vi "Vision Tracking.vi"(8 "error in (no error)":errorcluster, 11 "Ideal Target Height (in)":i32) -> (2 "Distance (ft)":dbl, 3 "X-Value of Target (px)":dbl)   [LabVIEW 2016]
uses:
  <vilib>/Rock Robotics/WPI/Camera/WPI_CameraSettings Read MJPG.ctl
  <vilib>/Rock Robotics/WPI/Camera/WPI_CameraImageSize.ctl
  2017 Robot Project/Vision Support Code/Camera Types.ctl
  <vilib>/Rock Robotics/WPI/Camera/WPI_CameraExposure Values.ctl
  <vilib>/Rock Robotics/WPI/Camera/WPI_CameraWhite Balance Values.ctl
  <vilib>/vision/NI_Vision_Development_Module.lvlib
panel:
  in  "Line Border":cluster{"Top":dbl, "Bottom":dbl}={"Top"=6.0, "Bottom"=1.0}
  in  "Use Calibration":bool=TRUE
  out "Instructions:":string="Use Source to load image files from a directory, or use a USB or IP camera connected to your laptop. Use Camera Settings 1 and 2 to achieve a dark image with bright and colorful stripes.\nLED Color can encoded as HSL or related color modes. Calibrate to the same color as the strips being reflected to the camera.\nClick and draw a line in Original Image to auto-calibrate the LED Color. You may want to widen and tweak Sat and Val by hand.\nThe Annotate button affects drawing a rectangle around the stripes and labeling it with a distance in ft. Distance relies on knowing the Camera Type and lens calibration (it looks up the lens view angle).\n\nAdjust Score Cutoff to make the code more or less picky. If the color is not very unique, you may need to increase the number of particles considered. The diagram uses a Size Limit to ignore colored things that are too small. You may need to adjust it if you are targetting from far away.\n\nResults give you the distance to the target, the center and box in a normalized (-1 to 1) and pixel coordinates.\n\nBe sure to read about setting camera exposure and brightness to help simplify your image and acquire color saturated images.\n\nThere are lots of comments on the diagram to explain the code."
  in  "Color Mode":u16(ring)=3 items=["RGB", "HSL", "HSV", "HSI"]
  in  "Particles":dbl=5.0
  in  "Score Cutoff %":dbl=70.0
  in  "Std Devs for Calibration":cluster{"H":dbl, "S":dbl, "V":dbl}={"H"=4.0, "S"=6.0, "V"=6.0}
  in  "Camera Type":T1=enum."MS HD3000 square"
  in  "image files":string[](array[string])
  out "Results":T2 {"Score" format="%#_3g"; "Pixels"."Rectangle"."Numeric 5" format="%#_3g"; "Pixels"."Rectangle"."Numeric 3" format="%#_3g"; "Pixels"."Rectangle"."Numeric 2" format="%#_3g"; "Pixels"."Rectangle"."Numeric" format="%#_3g"; "Normalized"."Rectangle"."Numeric 5" format="%#_2g"; "Normalized"."Rectangle"."Numeric 3" format="%#_2g"; "Normalized"."Rectangle"."Numeric 2" format="%#_2g"; "Normalized"."Rectangle"."Numeric" format="%#_2g"; "Normalized"."Center"."?" format="%#_3g"; "Normalized"."Center"."?" format="%#_3g"; "Distance (ft)" format="%#_3g"}
  in  "Source":enum32{"Files", "Camera"}(tab)
  in  "Images":i32(listbox)
  in  "Folder Location":path=path "C:/Program Files (x86)/National Instruments/LabVIEW 2016/examples/FRC/roboRIO/Vision/2017 Vision Example/Sample Images/LED Boiler"
  in  "Camera Settings":T3={"fps"=20, "compression"=30, "Image Size"=enum."320x240", "Config Shown"=FALSE}
  in  "Camera Address":string="USB 1"
  in  "Camera Settings 2":T7={"Exposure"=enum."Auto", "Exposure (%)"=50.0, "Brightness"=50, "White Balance"=enum."Auto", "Color Temp (K)"=0.0} {"Brightness" min=0 max=100}
  in  "Annotate":bool=TRUE
  out "Qualified Particles":i32
  in  "LED Color":T8={"Hue"={107.81818389892578, 139.81818389892578}, "Sat"={176.07142857142858, 255.0}, "Val"={40.53571428571429, 255.0}} {"Hue" scale=0.0..255.0 scale format="%#_3g"}
  out "Mask":T9(plugin-control)
  out "Original Image":T9(plugin-control)
  # "Legend:\n    Rectangle\n       Green - Good target, distance ft\n       Red - Bad target\n    Orange Text - Score in %"
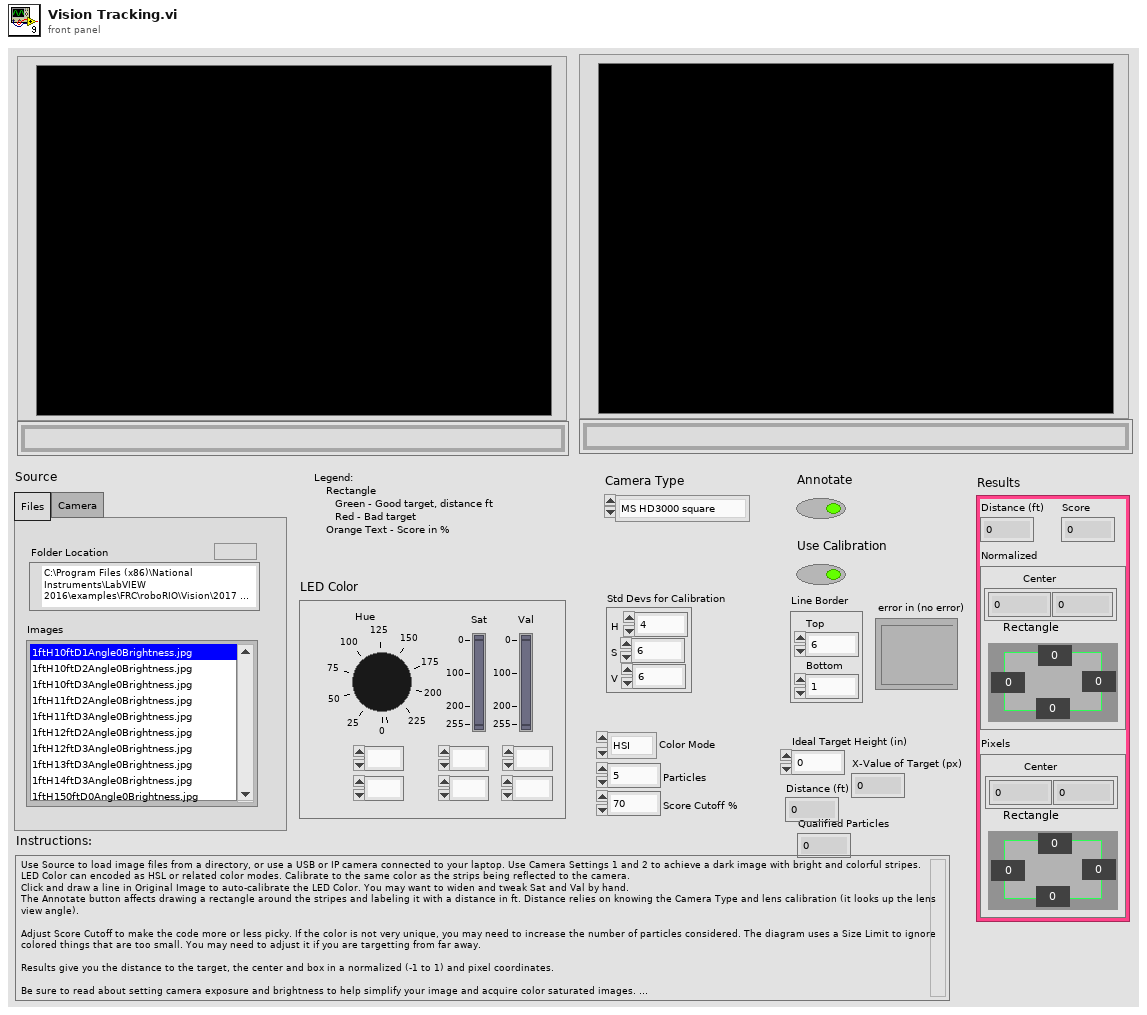
[diagram p1: front panel]
types:
  T1 = typedef "Camera Types.ctl" = enum16{"206", "1011", "1013", "MS HD3000 square", "MS HD3000 640x480"}
  T2 = cluster{"Distance (ft)":dbl, "Score":dbl, "Normalized":cluster{"Center":cluster{dbl, dbl}, "Rectangle":cluster{"Numeric":dbl, "Numeric 2":dbl, "Numeric 3":dbl, "Numeric 5":dbl}}, "Pixels":cluster{"Center":cluster{dbl, dbl}, "Rectangle":cluster{"Numeric":dbl, "Numeric 2":dbl, "Numeric 3":dbl, "Numeric 5":dbl}}}
  T3 = typedef "WPI_CameraSettings Read MJPG.ctl" = cluster{"fps":i32, "compression":i32, "Image Size":T4, "Config Shown":bool}
  T4 = typedef "WPI_CameraImageSize.ctl" = enum16{"640x480", "320x240", "160x120", "Custom"}
  T5 = typedef "WPI_CameraExposure Values.ctl" = enum16{"Auto", "Flicker-free 50 Hz", "Flicker-free 60 Hz", "Hold current", "Custom"}
  T6 = typedef "WPI_CameraWhite Balance Values.ctl" = enum16{"Auto", "Fixed indoor", "Fixed outdoor 1", "Fixed outdoor 2", "Fixed fluorescent 1", "Fixed fluorescent 2", "Hold current", "Custom"}
  T7 = cluster{"Exposure":T5, "Exposure (%)":dbl, "Brightness":i32, "White Balance":T6, "Color Temp (K)":dbl}
  T8 = cluster{"Hue":cluster{dbl, dbl}, "Sat":cluster{dbl, dbl}, "Val":cluster{dbl, dbl}}
  T9 = typedef "IMAQ Image.ctl" = refnum<image>
  T10 = typedef "Image Type" = u32
  T11 = typedef "Particle Parameters" = i32
  T12 = cluster{cluster{dbl, dbl}, cluster{dbl, dbl}, cluster{dbl, dbl}}
  T13 = cluster{"Left":dbl, "Top":dbl, "Right":dbl, "Bottom":dbl}
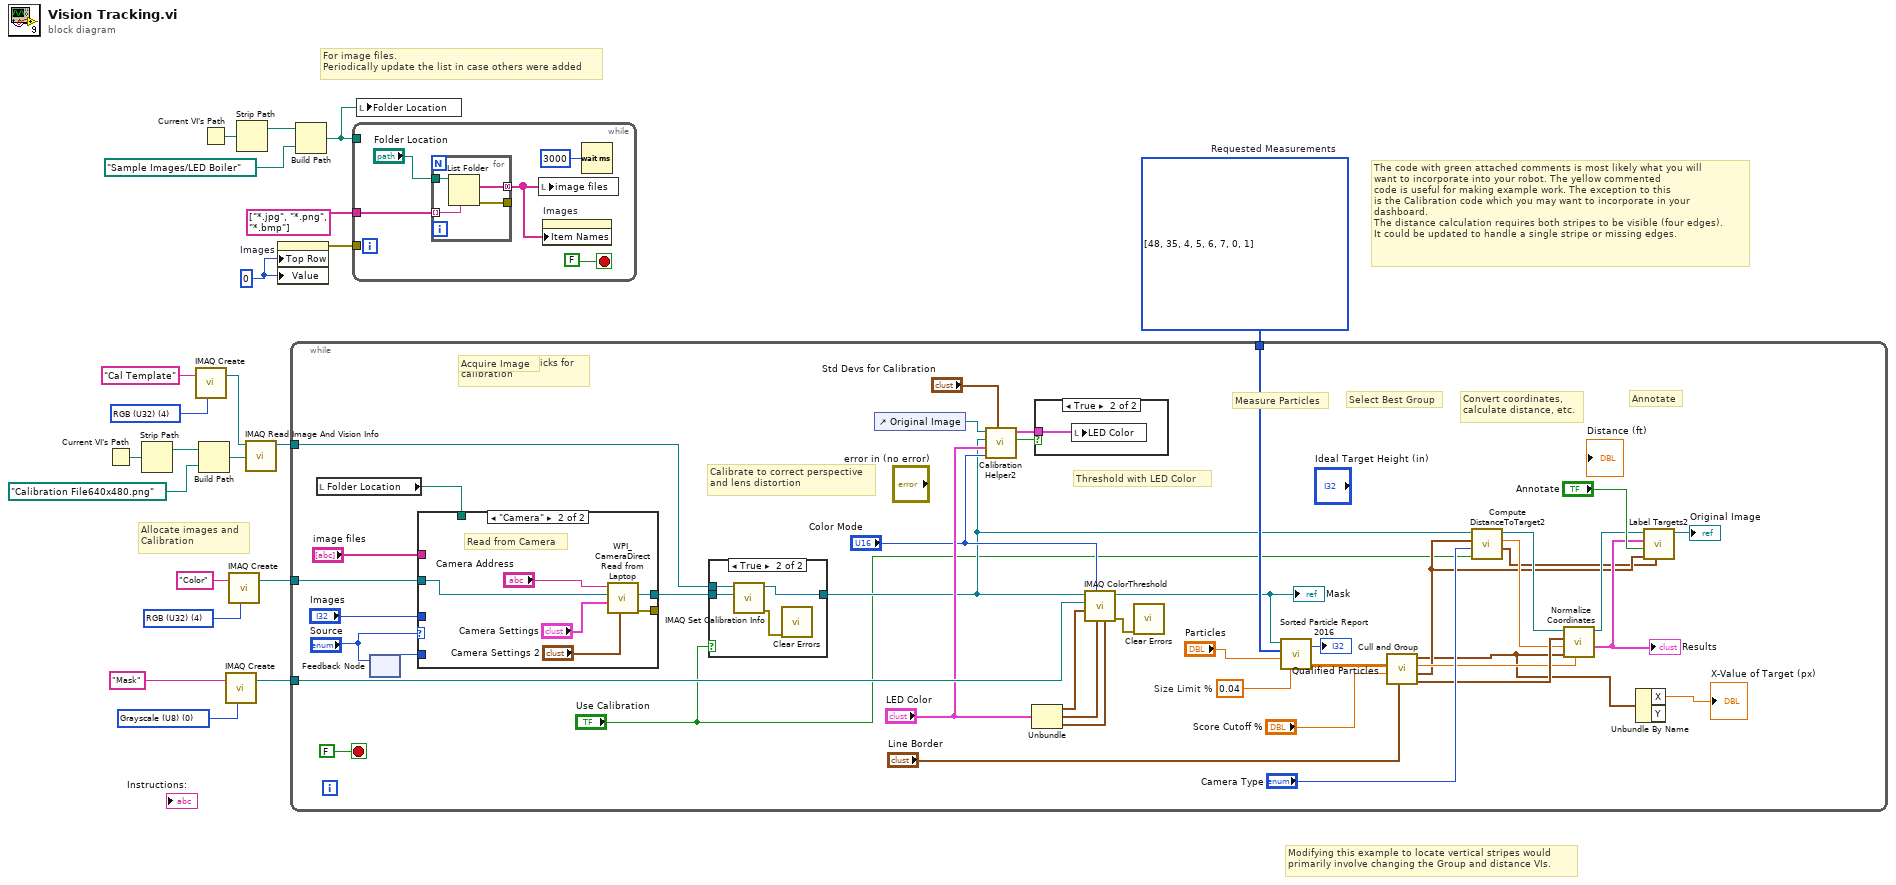
[diagram p0: block diagram]
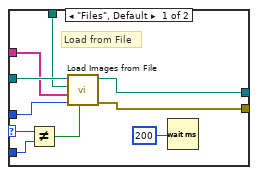
[diagram p4: hidden frame]
diagram:
  w8 = T10 4 items=["Grayscale (U8)", "Grayscale (I16)", "Grayscale (SGL)", "Complex (CSG)", "RGB (U32)", "HSL (U32)", "RGB (U64)", "Grayscale (U16)"] ("Image Type")
  w11 = u32 0 ("milliseconds to wait")
  w17 = T11[] [48, 35, 4, 5, 6, 7, 0, 1] items=["Center of Mass X", "Center of Mass Y", "First Pixel X", "First Pixel Y", "Bounding Rect Left", "Bounding Rect Top", "Bounding Rect Right", "Bounding Rect Bottom", "Max Feret Diameter Start X", "Max Feret Diameter Start Y", "Max Feret Diameter End X", "Max Feret Diameter End Y", "Max Horiz. Segment Length Left", "Max Horiz. Segment Length Right", "Max Horiz. Segment Length Row", "-", "Bounding Rect Width", "Bounding Rect Height", "Bounding Rect Diagonal", "Perimeter", "Convex Hull Perimeter", "Holes' Perimeter", "Max Feret Diameter", "Equivalent Ellipse Major Axis", "Equivalent Ellipse Minor Axis", "Equivalent Ellipse Minor Axis (Feret)", "Equivalent Rect Long Side", "Equivalent Rect Short Side", "Equivalent Rect Diagonal", "Equivalent Rect Short Side (Feret)", "Average Horiz. Segment Length", "Average Vert. Segment Length", "Hydraulic Radius", "Waddel Disk Diameter", "-", "Area", "Holes' Area", "Particle & Holes' Area", "Convex Hull Area", "Image Area", "-", "Number of Holes", "Number of Horiz. Segments", "Number of Vert. Segments", "-", "Orientation", "Max Feret Diameter Orientation", "-", "% Area/Image Area", "% Area/(Particle & Holes' Area)", "Ratio of Equivalent Ellipse Axes", "Ratio of Equivalent Rect Sides", "-", "Elongation Factor", "Compactness Factor", "Heywood Circularity Factor", "Type Factor", "-", "Sum X", "Sum Y", "Sum XX", "Sum XY", "Sum YY", "Sum XXX", "Sum XXY", "Sum XYY", "Sum YYY", "-", "Moment of Inertia XX", "Moment of Inertia XY", "Moment of Inertia YY", "Moment of Inertia XXX", "Moment of Inertia XXY", "Moment of Inertia XYY", "Moment of Inertia YYY", "Norm. Moment of Inertia XX", "Norm. Moment of Inertia XY", "Norm. Moment of Inertia YY", "Norm. Moment of Inertia XXX", "Norm. Moment of Inertia XXY", "Norm. Moment of Inertia XYY", "Norm. Moment of Inertia YYY", "Hu Moment 1", "Hu Moment 2", "Hu Moment 3", "Hu Moment 4", "Hu Moment 5", "Hu Moment 6", "Hu Moment 7"]  # Requested Measurements
  w20 = T10 0 items=["Grayscale (U8)", "Grayscale (I16)", "Grayscale (SGL)", "Complex (CSG)", "RGB (U32)", "HSL (U32)", "RGB (U64)", "Grayscale (U16)"] ("Image Type")
  w21 = T10 4 items=["Grayscale (U8)", "Grayscale (I16)", "Grayscale (SGL)", "Complex (CSG)", "RGB (U32)", "HSL (U32)", "RGB (U64)", "Grayscale (U16)"] ("Image Type")
  # "Modifying this example to locate vertical stripes would\nprimarily involve changing the Group and distance VIs."
  # "The code with green attached comments is most likely what you will\nwant to incorporate into your robot. The yellow commented\ncode is useful for making example work. The exception to this\nis the Calibration code which you may want to incorporate in your\ndashboard.\nThe distance calculation requires both stripes to be visible (four edges).\nIt could be updated to handle a single stripe or missing edges."
  # "For image files.\nPeriodically update the list in case others were added"
  # "Allocate images and\nCalibration"
  n1 = Current VI's Path() -> (path=w4:path)
  n2 = Strip Path(path=w4) -> (stripped path=w1:path)  [unwired: 1 out]
  n3 = call "IMAQ Create"("Image Name"="Cal Template", "Image Type"=w8) -> ("New Image"=w6:T9)  [unwired: 2 in, 2 out]
  n4 = Build Path(base path=w1, name or relative path=path "Calibration File640x480.png" ("Folder Location")) -> (appended path=w3:path)
  n5 = Current VI's Path() -> (path=w16:path)
  n6 = call "IMAQ Create"("Image Name"="Mask", "Image Type"=w20) -> ("New Image"=w18:T9)  [unwired: 2 in, 2 out]
  n7 = call "IMAQ Create"("Image Name"="Color", "Image Type"=w21) -> ("New Image"=w9:T9)  [unwired: 2 in, 2 out]
  n8 = Strip Path(path=w16) -> (stripped path=w14:path)  [unwired: 1 out]
  n9 = call "IMAQ Read Image And Vision Info"("File Path"=w3, "Image"=w6) -> ("Image Out"=w5:T9)  [unwired: 7 in, 2 out]
  n10 = property on="Images" class="LstBox (strict)"("Top Row"=w11, "Value"=w11) -> (error out=w12:errorcluster)  [unwired: 2 in, 1 out]
  n11 = while {
    tunnel: w9 -> [w64]
    tunnel: w18 -> [w62]
    tunnel: w17 -> [w58]
    tunnel: w5 -> [w27]
    stop <- FALSE stop-if-true
    w56 = 0.04  # Size Limit %
    # "Calibrate to correct perspective\nand lens distortion"
    # "Handle Mouse clicks for\ncalibration"
    # "Measure Particles"
    # "Convert coordinates,\ncalculate distance, etc."
    # "Annotate"
    # "Select Best Group"
    # "Threshold with LED Color"
    # "Acquire Image"
    n12 = local read "Folder Location"() -> (w46:path)
    n13 = feedback-in #1("Source") -> ()
    n14 = feedback #1() -> (w44:enum32{"Files", "Camera"})  [unwired: 1 in]
    n15 = case shown="\"Camera\"" "Source" {
      selector: "Source" -> [w74 _]
      tunnel: [w80 w87] -> _
      tunnel: [w81 w86] -> w28
      tunnel: w64 -> [w79 w85]
      tunnel: "image files" -> [w76 _]
      tunnel: "Images" -> [w78 _]
      tunnel: w46 -> [w77 _]
      tunnel: w44 -> [w73 _]
      frame "Files", Default {
        # "Load from File"
        n16 = Not Equal?(x=w74, y=w73) -> (x != y?=w72:bool)
        n17 = call "Load Images from File.vi"("Force Load"=w72, "Images"=w78, "image files"=w76, "Folder Location"=w77, "Refnum in"=w79) -> ("error out"=w80:errorcluster, "Refnum out"=w81:T9)  [unwired: 5 in]
        n18 = Wait (ms)(milliseconds to wait=u32 200 ("delay (ms)")) -> ()  [unwired: 1 out]
      }
      frame "Camera" {
        # "Read from Camera"
        n19 = call <vilib>:"WPI_CameraDirect Read from Laptop.vi"("Camera Settings 2"="Camera Settings 2", "Camera Settings"="Camera Settings", "Image"=w85, "address"="Camera Address") -> ("error out"=w87:errorcluster, "Image Out"=w86:T9)  [unwired: 6 in]
      }
    }
    n20 = case shown="True" "Use Calibration" {
      tunnel: [w66 w70] -> w29
      tunnel: w28 -> [w66 w69]
      tunnel: w27 -> [_ w68]
      frame False {
      }
      frame True {
        n21 = call "IMAQ Set Calibration Info"("Image Dst"=w69, "Image Src"=w68) -> ("error out"=w67:errorcluster, "Calibrated Image"=w70:T9)  [unwired: 8 in]
        n22 = call <vilib>:"Clear Errors.vi"("error in (no error)"=w67) -> ()  [unwired: 5 in, 2 out]
      }
    }
    n23 = control-ref of="Original Image"() -> (w51:refnum<vi>)
    n24 = call "Calibration Helper2.vi"("Std Devs"="Std Devs for Calibration", "Color Mode"="Color Mode", "Color Components"="LED Color", "Image"=w29, "Image Ctl Refnum"=w51) -> ("Changed"=w50:bool, "output color"=w49:T12)  [unwired: 5 in]
    n25 = Unbundle("LED Color") -> ("Hue"=w61:cluster{dbl, dbl}, "Sat"=w60:cluster{dbl, dbl}, "Val"=w59:cluster{dbl, dbl})
    n26 = case shown="True" w50 {
      tunnel: w49 -> [_ w71]
      frame False {
      }
      frame True {
        n27 = local write "LED Color"(w71) -> ()
      }
    }
    n28 = call "IMAQ ColorThreshold"("Blue or Luma or Val or Inten Range"=w59, "Green or Sat Range"=w60, "Color Mode"="Color Mode", "Red or Hue Range"=w61, "Image Dst"=w62, "Image Src"=w29) -> ("error out"=w52:errorcluster, "Image Dst Out"=w41:T9)  [unwired: 4 in]
    "Mask" <- w41
    n29 = call <vilib>:"Clear Errors.vi"("error in (no error)"=w52) -> ()  [unwired: 5 in, 2 out]
    n30 = call "Sorted Particle Report 2016.vi"("Min Area Size %"=w56, "Particle Count Limit"="Particles", "Pixel Measurements"=w58, "Image in"=w41) -> ("Sorted Data"=w43:dbl[][], "Particles"=→"Qualified Particles":i32)
    n31 = call "Cull and Group.vi"("Line Border"="Line Border", "Score Cutoff"="Score Cutoff %", "Sorted Data"=w43) -> ("Rect"=w39:T13, "Line"=w31:T13, "Score"=w34:dbl, "Center"=w24:cluster{"X":dbl, "Y":dbl})  [unwired: 5 in]
    n32 = call "Compute DistanceToTarget2.vi"("Calibrated"="Use Calibration", "Camera Type"="Camera Type", "Line"=w31, "Image Src"=w29) -> ("Edges"=w30:cluster{"X":sgl, "Y":sgl}[], "Distance (ft)"=w38:dbl, "Image Dst Out"=w37:T9)  [unwired: 5 in]
    n33 = call "Normalize Coordinates.vi"("Score"=w34, "Center"=w24, "Distance"=w38, "Bounding box"=w39, "Image in"=w37) -> ("Results"=w35:T2, "Image out"=w36:T9)  [unwired: 5 in]
    "Results" <- w35
    n34 = Unbundle By Name(w24) -> ("X"=→"X-Value of Target (px)":dbl)  [unwired: 1 out]
    n35 = call "Label Targets2.vi"("Edges"=w30, "Line"=w31, "Annotate"="Annotate", "Results"=w35, "Image in"=w36) -> ("Image out"=→"Original Image":T9)  [unwired: 6 in]
  }
  n36 = Build Path(base path=w14, name or relative path=path "Sample Images/LED Boiler" ("Folder Location")) -> (appended path=w13:path)
  n37 = while {
    tunnel: w13 -> [_]
    tunnel: w12 -> [_]
    tunnel: string[] ["*.jpg", "*.png", "*.bmp"] -> [w88]
    stop <- FALSE stop-if-true
    n38 = for {
      tunnel: [w96] -> w90 mode=concatenating
      tunnel: "Folder Location" -> [w95]
      tunnel: [w94] -> _
      tunnel: w88 -> [w93] mode=indexing
      n39 = List Folder(path=w95, pattern=w93) -> (filenames=w96:string[], error out=w94:errorcluster)  [unwired: 2 in, 2 out]
    }
    n40 = local write "image files"(w90) -> ()
    n41 = property on="Images" class="LstBox (strict)"("Item Names"=w90) -> ()  [unwired: 2 in, 2 out]
    n42 = Wait (ms)(milliseconds to wait=u32 3000) -> ()  [unwired: 1 out]
  }
  n43 = local write "Folder Location"(w13) -> ()
